vi "Cpeak_manual.vi"() -> ()   [LabVIEW 2019, in "Prueba09.lvclass"]
uses:
  Prueba09/Prueba09.lvclass
  Instrumento/DS360/DS360.lvclass
panel:
  in  "knobFrec":dbl(knob)=1.0 min=1.0 max=3.0 scale=1.0..3.0
  out "error out":errorcluster
  in  "error in (no error)":errorcluster
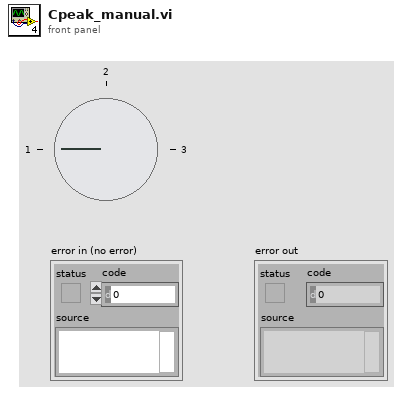
[diagram p1: front panel]
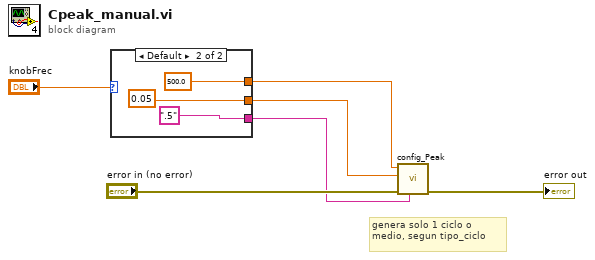
[diagram p0: block diagram]
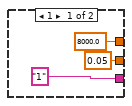
[diagram p2: hidden frame]
diagram:
  # "genera solo 1 ciclo o medio, segun tipo_ciclo"
  n1 = case shown="Default" "knobFrec" {
    tunnel: ["1" ".5"] -> w1
    tunnel: [8000.0 ("frec") 500.0 ("frec")] -> w3
    tunnel: [0.05 ("frec") 0.05 ("frec")] -> w2
    frame 1 {
    }
    frame Default {
    }
  }
  n2 = call "config_Peak.vi"("tipo_ciclo"=w1, "error in (no error)"="error in (no error)", "Amplitud (Vrms)"=w2, "Frec (Hz)"=w3) -> ("error out"=→"error out":errorcluster)  [unwired: 6 in, 1 out]
